vi "PicoScope6000GetValuesBulk.vi"(5 "Segment Range":T1 {"toSegmentIndex" format="%.4p"; "fromSegmentIndex" format="%.4p"}, 7 "Buffer and Transfer Settings":T2 {"Down-Sample Mode" items=["RAW none", "None", "Aggregate", "Decimate", "Average"]; "Down Sample Ratio" step=1; "Samples" format="%_6p"}, 8 "error in (no error)":errorcluster, 11 "handle in":i16) -> (0 "error out":errorcluster, 3 "handle out":i16, 4 "overflow":i16[](array[numeric]) format="%010b", 6 "noOfSamples":u64)   [LabVIEW 2009]
doc: "Calls ps5000aGetValuesOverlapped"
uses:
  ps6000.dll
  shared/Segment Range.ctl
  shared/Buffer and Transfer Settings.ctl
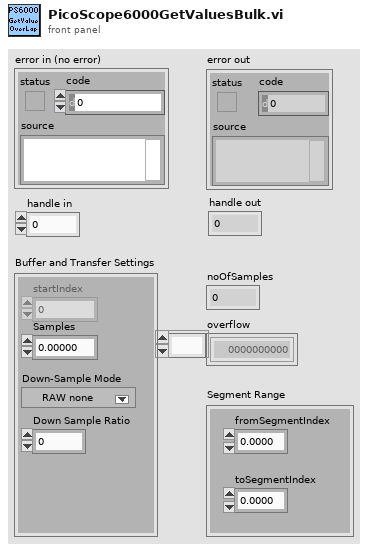
[diagram p1: front panel]
types:
  T1 = typedef "Segment Range.ctl" = cluster{"fromSegmentIndex":u64, "toSegmentIndex":u64}
  T2 = typedef "Buffer and Transfer Settings.ctl" = cluster{"startIndex":u64, "Samples":u64, "Down Sample Ratio":u64, "Down-Sample Mode":u32}
  T3 = cluster{"status":bool, "code":u32, "source":string}
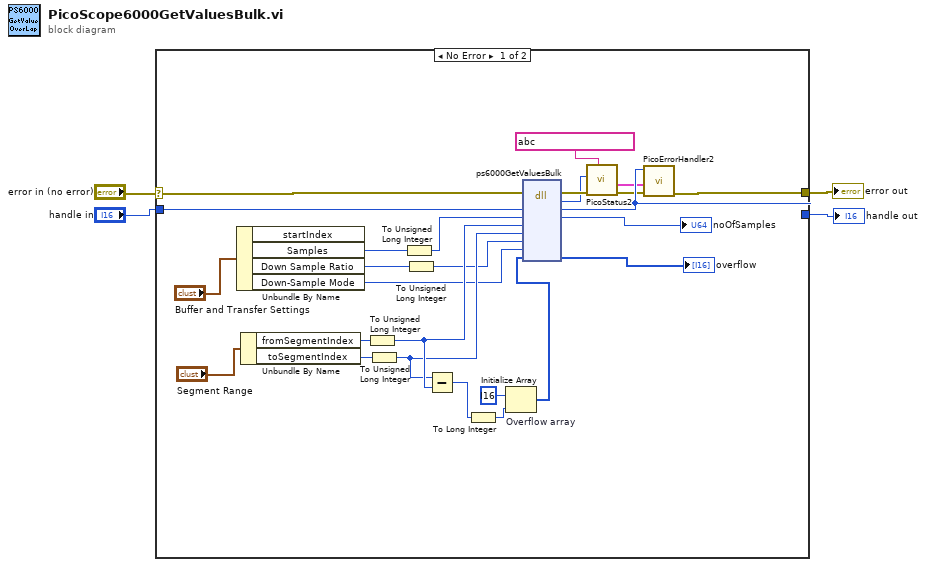
[diagram p0: block diagram]
diagram:
  n1 = case shown="No Error" "error in (no error)" {
    selector: "error in (no error)" -> [w29 w31]
    tunnel: "handle in" -> [w28 w32]
    tunnel: [w26 w32] -> w4
    tunnel: [w27 w31] -> w3
    frame #0 {
      n2 = Unbundle By Name("Buffer and Transfer Settings") -> ("Samples"=w18:u64, "Down Sample Ratio"=w17:u64, "Down-Sample Mode"=w5:u32)  [unwired: 1 out]
      n3 = Unbundle By Name("Segment Range") -> ("fromSegmentIndex"=w15:u64, "toSegmentIndex"=w16:u64)
      n4 = To Unsigned Long Integer(number=w15) -> (unsigned 32bit integer=w8:u32)
      n5 = To Unsigned Long Integer(number=w16) -> (unsigned 32bit integer=w7:u32)
      n6 = To Unsigned Long Integer(number=w18) -> (unsigned 32bit integer=w9:u32)
      n7 = To Unsigned Long Integer(number=w17) -> (unsigned 32bit integer=w6:u32)
      n8 = Subtract(x=w7, y=w8) -> (x-y=w12:u32)
      n9 = To Long Integer(number=w12) -> (32bit integer=w13:i32)
      n10 = Initialize Array "Overflow array"(i16 ? ("element"), w13) -> (w11:i16[])
      n11 = dll-call lib="ps6000.dll" fn="ps6000GetValuesBulk" ("ps3000.dll:_ps3000_open_unit@0")(error in=w29, "handle"=w28, "noOfSamples"=w9, "fromSegmentIndex"=w8, "toSegmentIndex"=w7, "downSampleRatio"=w6, "downSampleRatioMode"=w5, "overflow"=w11) -> (error out=w22:errorcluster, "PICO_STATUS"=w19:u32, "handle"=w26:i16, "noOfSamples"=→"noOfSamples":u32, "overflow"=→"overflow":i16[])  [unwired: 6 in, 1 out]
      n12 = call "PicoStatus2.vi"("PICO source"=string ? ("source"), "Error in"=w22, "PICO STATUS"=w19) -> ("error out"=w23:errorcluster, "PICO_STATUS out"=w20:T3)  [unwired: 5 in]
      n13 = call "PicoErrorHandler2.vi"("error in (no error)"=w23, "PICO_STATUS in"=w20, "handle In"=w26) -> ("error out"=w27:errorcluster)  [unwired: 8 in]
    }
    frame #1 {
    }
  }
  "error out" <- w3
  "handle out" <- w4
